vi "svfa_Process FRF (NxM).vi"(0 "stimulus signals X [EUx]":waveform(dbl)[](array[waveform]), 1 "response signals Y [EUy]":waveform(dbl)[](array[waveform]), 2 "window":T9=1 items=["None"=0, "Hanning"=1, "Hamming"=2, "Blackman-Harris"=3, "Exact Blackman"=4, "Blackman"=5, "Flat Top"=6, "4 Term B-Harris "=7, "7 Term B-Harris"=8, "Low Sidelobe"=9, "Force - Exponential"=10, "Blackman Nuttall"=11, "Triangle"=30, "Bartlett-Hanning"=31, "Bohman"=32, "Parzen"=33, "Welch"=34, "Kaiser"=60, "Dolph-Chebyshev"=61, "Gaussian"=62], 3 "force/exp settings":T8={"force window [%]"=50.0, "exp window [%]"=10.0} {"exp window [%]" min=0.0 max=100.0 format="%.2f"; "force window [%]" min=0.0 max=100.0 format="%.2f"}, 4 "averaging parameters":T12={"averaging mode"=enum."No averaging", "weighting mode"=enum."Linear", "number of averages"=10, "linear mode"=enum."Auto restart"}, 5 "error in (no error)":errorcluster, 7 "processing control":T10(ring), 9 "FRF mode":enum16{"H1", "H2", "H3"}(ring), 11 "spectra info in":T1[][](array[typedef]) {"x-axis units" items=["Time (s)"=0, "Frequency-CB (Hz)"=1, "Frequency-CPB (Hz)"=1248, "Frequency-Arbitrary (Hz)"=2357, "Quefrency (s)"=2, "Revolutions (rev)"=3, "Order"=4, "Speed (RPM)"=11, "Speed (rad/s)"=21, "Index"=65535]; "weighting filter" items=["Linear", "A-weighting", "B-weighting", "C-weighting", "ITU-R 468-4", "Dolby", "CCITT", "C-message", "Wb", "Wc", "Wd", "We", "Wf", "Wh", "Wj", "Wk", "Wm", "AES17 20 kHz lowpass", "AES17 40 kHz lowpass", "AES17 20 kHz highpass", "AES17 40 kHz highpass"]; "dB reference [EU]" format="%.2f"; "engineering units" items=["custom..."=0, "V"=1, "A"=21, "C"=30, "pC"=31, "s"=32, "-"=29, "Pa"=2, "N"=20, "g"=3, "m/s^2"=4, "m/s"=5, "m"=6, "mm/s"=12, "mm"=13, "micron/s"=14, "micron"=15, "in/s^2"=7, "in/s"=8, "in"=9, "mil/s"=10, "mil"=11, "rad/s^2"=16, "rad/s"=17, "rad"=18, "deg/s^2"=26, "deg/s"=27, "deg"=28, "RPM"=22, "cycle/s^2"=23, "Hz"=24, "cycle"=25, "strain"=19]; "spectral info"."window" items=["None "=0, "Hanning"=1, "Hamming"=2, "Blackman-Harris"=3, "Exact Blackman"=4, "Blackman"=5, "Flat Top"=6, "4 Term B-Harris "=7, "7 Term B-Harris"=8, "Low Sidelobe"=9, "Force - Exponential"=10, "Gaussian"=62]}) -> (8 "stimulus signals X [EUx] 2":waveform(dbl)[](array[waveform]), 10 "response signals Y [EUy] 2":waveform(dbl)[](array[waveform]), 12 "averages completed":dbl format="%.2f", 13 "processing control":T10(ring), 14 "complex responses [EUy/EUx]":T7(array[cluster]) {"complex spectrum" format="%.2f"; "df" format="%.2f"; "f0" format="%.2f"}, 16 "coherence":T11(array[cluster]) {"coherence" format="%.2f"; "df" format="%.2f"; "f0" format="%.2f"}, 17 "averaging done":bool, 18 "spectra info out":T1[][](array[typedef]) {"x-axis units" items=["Time (s)"=0, "Frequency-CB (Hz)"=1, "Frequency-CPB (Hz)"=1248, "Frequency-Arbitrary (Hz)"=2357, "Quefrency (s)"=2, "Revolutions (rev)"=3, "Order"=4, "Speed (RPM)"=11, "Speed (rad/s)"=21, "Index"=65535]; "weighting filter" items=["Linear", "A-weighting", "B-weighting", "C-weighting", "ITU-R 468-4", "Dolby", "CCITT", "C-message", "Wb", "Wc", "Wd", "We", "Wf", "Wh", "Wj", "Wk", "Wm", "AES17 20 kHz lowpass", "AES17 40 kHz lowpass", "AES17 20 kHz highpass", "AES17 40 kHz highpass"]; "dB reference [EU]" format="%.2f"; "engineering units" items=["custom..."=0, "V"=1, "A"=21, "C"=30, "pC"=31, "s"=32, "-"=29, "Pa"=2, "N"=20, "g"=3, "m/s^2"=4, "m/s"=5, "m"=6, "mm/s"=12, "mm"=13, "micron/s"=14, "micron"=15, "in/s^2"=7, "in/s"=8, "in"=9, "mil/s"=10, "mil"=11, "rad/s^2"=16, "rad/s"=17, "rad"=18, "deg/s^2"=26, "deg/s"=27, "deg"=28, "RPM"=22, "cycle/s^2"=23, "Hz"=24, "cycle"=25, "strain"=19]; "spectral info"."window" items=["None "=0, "Hanning"=1, "Hamming"=2, "Blackman-Harris"=3, "Exact Blackman"=4, "Blackman"=5, "Flat Top"=6, "4 Term B-Harris "=7, "7 Term B-Harris"=8, "Low Sidelobe"=9, "Force - Exponential"=10, "Gaussian"=62]}, 19 "error out":errorcluster)   [LabVIEW 2017]
uses:
  <vilib>/addons/_NISVFA/_Shared subVIs/Controls/svc_Window [Dual FFT].ctl
  <vilib>/addons/_NISVFA/_Shared subVIs/Controls/svc_Spectrum Info.ctl
  <vilib>/addons/_NISVFA/_Shared subVIs/Controls/svc_X-Axis Units.ctl
  <vilib>/addons/_NISVFA/_Shared subVIs/Controls/svc_Spectrum Type.ctl
  <vilib>/addons/_NISVFA/_Shared subVIs/Controls/svc_Engineering Units Text Ring.ctl
  <vilib>/addons/_NISVFA/_Shared subVIs/Controls/svc_Weighting Filter Text Ring.ctl
  <vilib>/addons/_NISVFA/_Shared subVIs/Controls/svc_Complimentary Spectrum Units.ctl
  <vilib>/addons/_NISVFA/_Shared subVIs/Windowing/svfa_Scaled Time Domain Window (N Ch).vi
  <vilib>/addons/_NISVFA/_Shared subVIs/Spectrum Averaging/svfa_Average Array (complex).vi
  <vilib>/addons/_NISVFA/_Shared subVIs/Spectrum Averaging/svfa_Average Array (real).vi
  <vilib>/addons/_NISVFA/_Shared subVIs/Windowing/svfa_Scaled Time Domain Window (1 Ch).vi
  <vilib>/addons/_NISVFA/_Shared subVIs/Windowing/svfa_Scaled Time Domain Window (Array).vi
  <vilib>/Analysis/4window.llb/Force Window.vi
  <vilib>/Analysis/4window.llb/Force Window (DBL).vi
  <vilib>/Analysis/4window.llb/Exponential Window.vi
  <vilib>/Analysis/4window.llb/Exponential Window (DBL).vi
  <vilib>/Utility/error.llb/Error Cluster From Error Code.vi
  <vilib>/Analysis/0measdsp.llb/Scaled Time Domain Window.vi
  <vilib>/Analysis/0measdsp.llb/Scaled Time Domain Window (DBL).vi
  <vilib>/addons/_NISVFA/_Spectrum Processing/subVIs/svfa_Spectrum Info Window to windowTd Type Def.vi
  <vilib>/addons/_NISVFA/_Shared subVIs/Common/svc_Window Parameters.vi
  <vilib>/addons/_NISVFA/_Shared subVIs/Common/svc_Get Window Info.vi
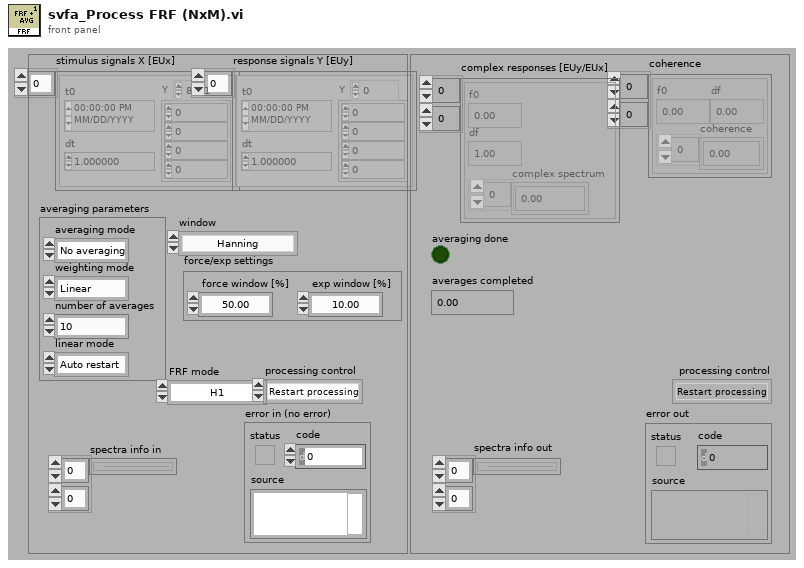
[diagram p1: front panel]
types:
  T1 = typedef "svc_Spectrum Info.ctl" = cluster{"channel name":string, "description":string, "x-axis units":T2, "spectral info":cluster{"spectrum type":T3, "linear/dB":enum16{"linear", "dB"}, "window":u16, "window size":i32, "FFT size":i32}, "engineering units":T4, "custom label":string, "dB reference [EU]":dbl, "peak units":enum16{"rms", "peak", "peak-peak"}, "weighting filter":T5, "spectral density?":bool, "unit label":string, "spectrum skewed?":bool, "complimentary spectrum units":T6}
  T2 = typedef "svc_X-Axis Units.ctl" = u16
  T3 = typedef "svc_Spectrum Type.ctl" = enum16{"FFT Spectrum [complex]", "Amplitude [Magnitude]", "Power [Magnitude^2]", "Cross Spectrum [complex]", "Frequency Response [Complex]"}
  T4 = typedef "svc_Engineering Units Text Ring.ctl" = u16
  T5 = typedef "svc_Weighting Filter Text Ring.ctl" = u16
  T6 = typedef "svc_Complimentary Spectrum Units.ctl" = enum16{"none", "radians", "degrees", "cycles", "imaginary"}
  T7 = cluster{"f0":dbl, "df":dbl, "complex spectrum":cdb[]}[][]
  T8 = cluster{"force window [%]":dbl, "exp window [%]":dbl}
  T9 = typedef "svc_Window [Dual FFT].ctl" = u32
  T10 = enum16{"Restart processing", "Continue processing", "Skip processing"}
  T11 = cluster{"f0":dbl, "df":dbl, "coherence":dbl[]}[][]
  T12 = cluster{"averaging mode":enum16{"No averaging", "Vector averaging", "RMS averaging", "Peak hold"}, "weighting mode":enum16{"Linear", "Exponential"}, "number of averages":u32, "linear mode":enum16{"One shot", "Auto restart"}}
  T13 = enum16{"No averaging", "Vector averaging", "RMS averaging", "Peak hold"}
  T14 = cluster{"f0":dbl, "df":dbl, "complex array":cdb[]}
  T15 = cluster{"f0":dbl, "df":dbl, "real FFT":dbl[]}[][]
  T16 = cluster{"f0":dbl, "df":dbl, "complex array":cdb[]}[]
  T17 = cluster{"f0":dbl, "df":dbl, "complex array":cdb[]}[][]
  T18 = cluster{"complex spectrum":cluster{"f0":dbl, "df":dbl, "complex spectrum":cdb[]}, "spectrum info":T1}
  T19 = cluster{"f0":dbl, "df":dbl, "complex spectrum":cdb[]}
  T20 = cluster{"f0":dbl, "df":dbl, "magnitude":dbl[]}[][]
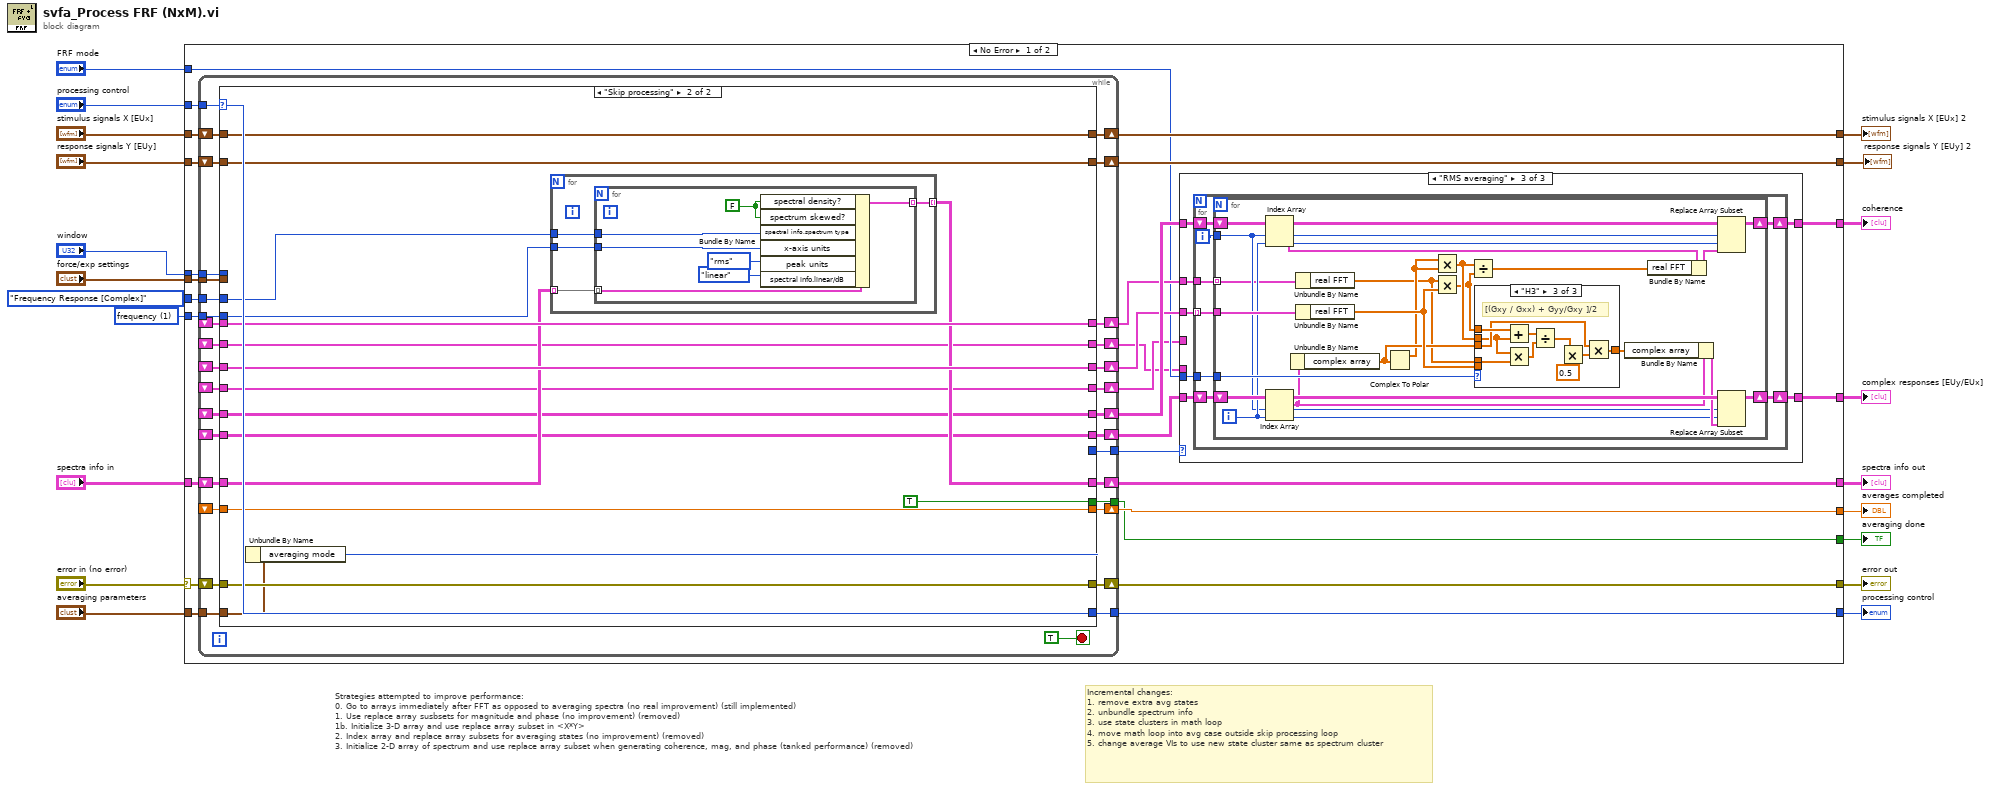
[diagram p0: block diagram]
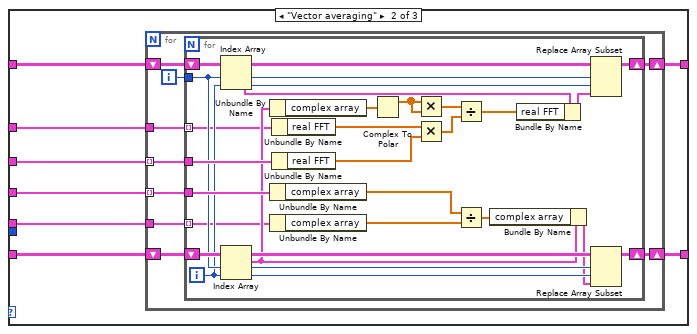
[diagram p3: hidden frame]
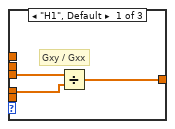
[diagram p4: hidden frame]
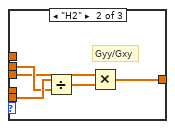
[diagram p5: hidden frame]
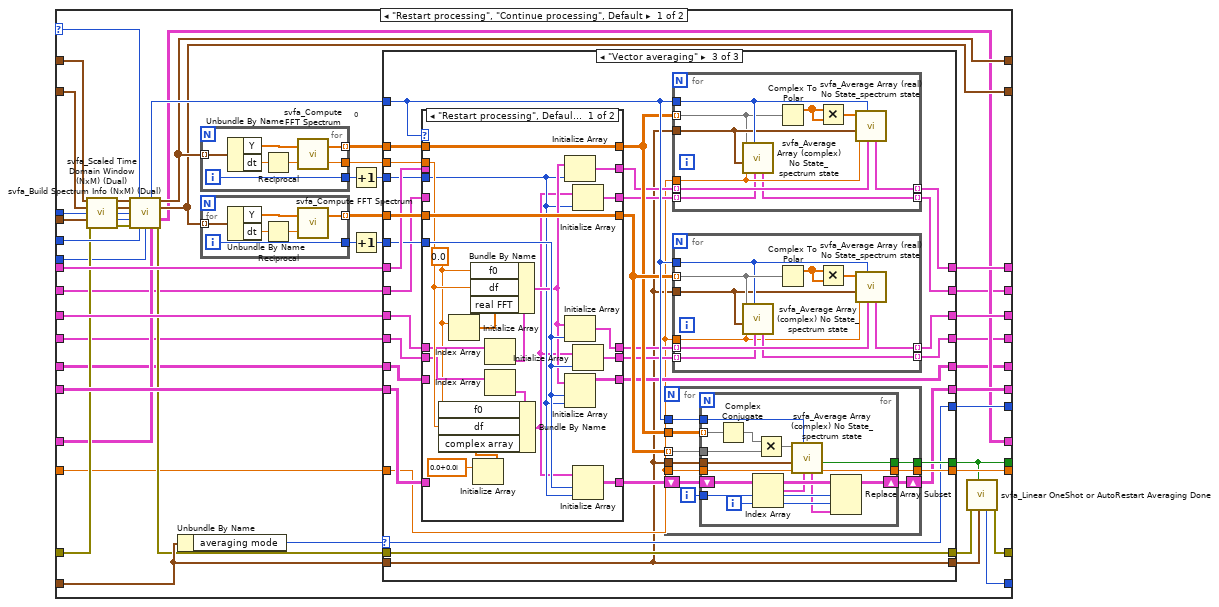
[diagram p6: hidden frame]
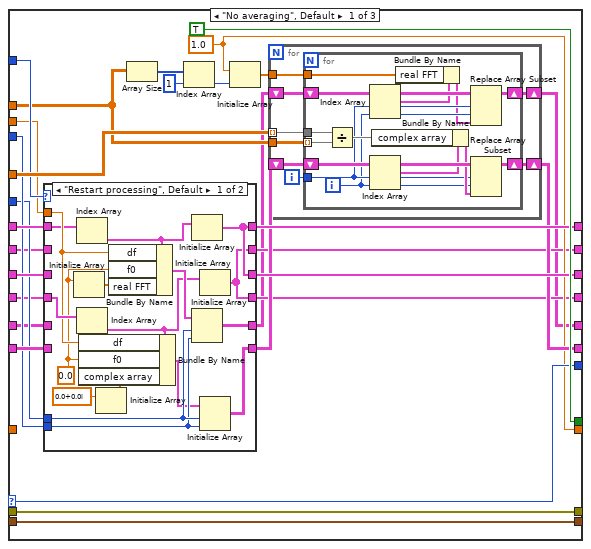
[diagram p7: hidden frame]
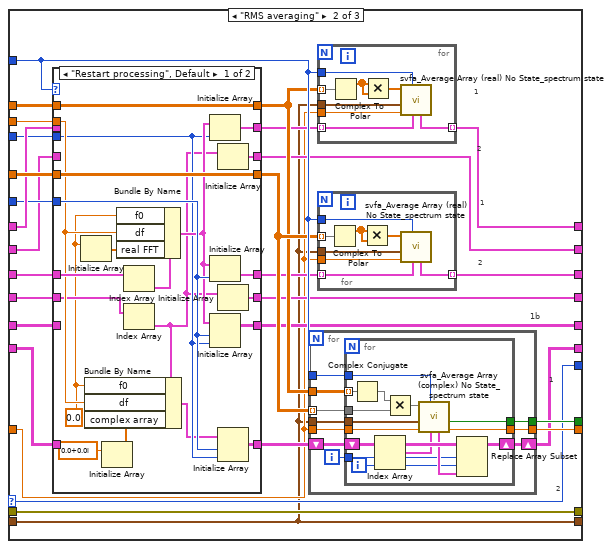
[diagram p9: hidden frame]
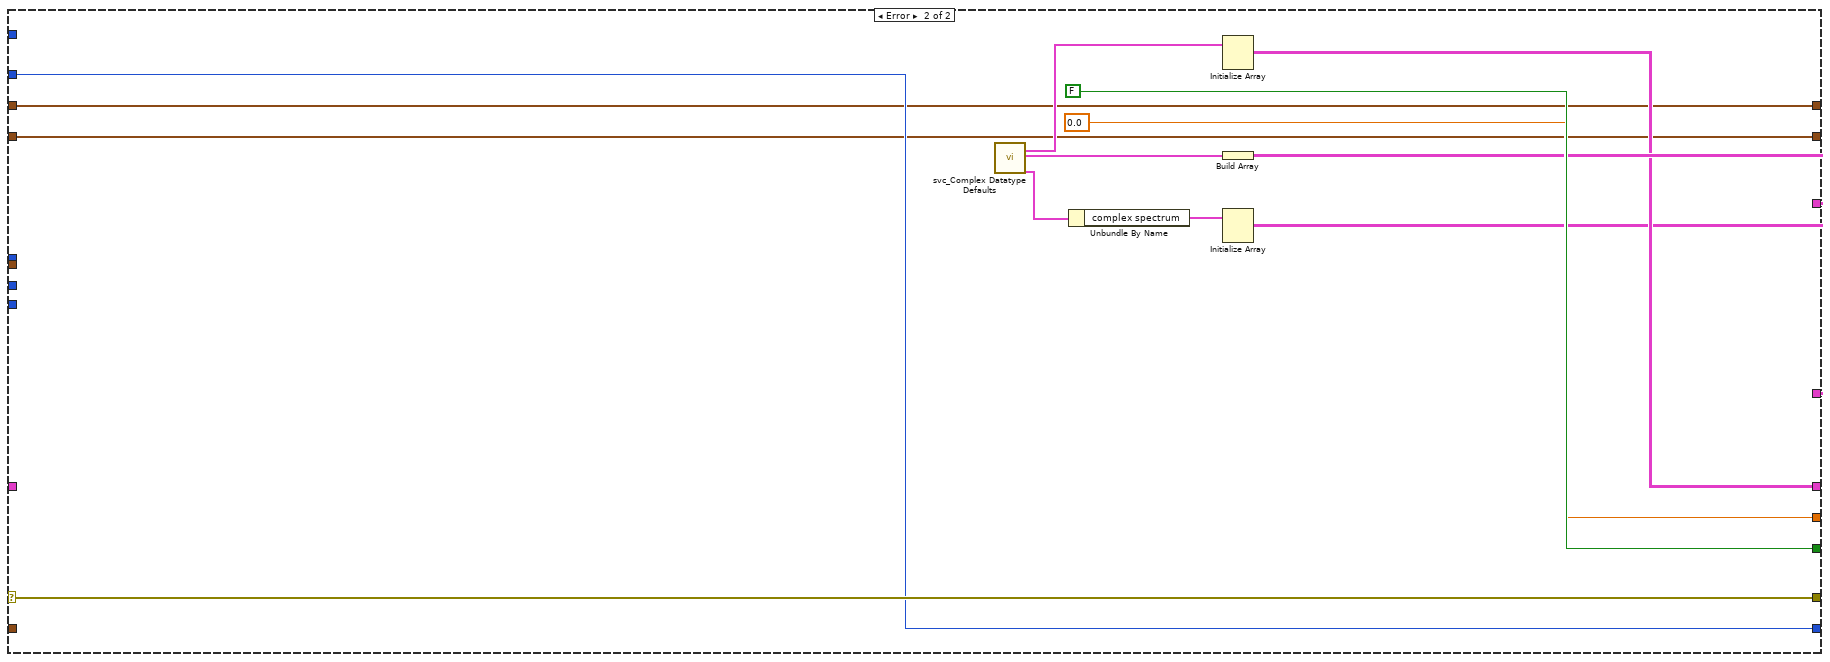
[diagram p12: hidden frame]
diagram:
  w6 = u16 1 items=["time"=0, "frequency"=1, "quefrency"=2, "revolutions"=3, "order"=4, "rpm"=11] ("x-axis units")
  # "Strategies attempted to improve performance:\n0. Go to arrays immediately after FFT as opposed to averaging spectra (no real improvement) (still implemented)\n1. Use replace array susbsets for magnitude and phase (no improvement) (removed)\n1b. Initialize 3-D array and use replace array subset in <X*Y>\n2. Index array and replace array subsets for averaging states (no improvement) (removed)\n3. Initialize 2-D array of spectrum and use replace array subset when generating coherence, mag, and phase (tanked performance) (removed)"
  # "Incremental changes:\n1. remove extra avg states\n2. unbundle spectrum info\n3. use state clusters in math loop\n4. move math loop into avg case outside skip processing loop\n5. change average VIs to use new state cluster same as spectrum cluster"
  n1 = case shown="No Error" "error in (no error)" {
    selector: "error in (no error)" -> [w44 w557]
    tunnel: [w38 w557] -> w20
    tunnel: "averaging parameters" -> [w47 _]
    tunnel: "stimulus signals X [EUx]" -> [w45 w546]
    tunnel: [w32 FALSE ("averaging done")] -> w16
    tunnel: [w46 0.0 ("averages completed")] -> w15
    tunnel: [w22 w547] -> w14
    tunnel: [w23 w552] -> w13
    tunnel: "FRF mode" -> [w26 _]
    tunnel: "processing control" -> [w43 w554]
    tunnel: [w39 w554] -> w10
    tunnel: "response signals Y [EUy]" -> [w42 w545]
    tunnel: "window" -> [w41 _]
    tunnel: "force/exp settings" -> [w40 _]
    tunnel: svc_Spectrum_Type."Frequency Response [Complex]" ("spectrum type") -> [w37 _]
    tunnel: w6 -> [w36 _]
    tunnel: [w35 w550] -> w5
    tunnel: [w34 w546] -> w4
    tunnel: [w33 w545] -> w3
    tunnel: "spectra info in" -> [w21 _]
    frame No Error {
      n2 = while {
        tunnel: [w168] -> w39
        tunnel: w40 -> [w169]
        tunnel: w41 -> [w170]
        tunnel: w43 -> [w165]
        tunnel: [w174] -> w32
        tunnel: w47 -> [w176]
        shift-right: [w164] -> w28
        shift-left: _ -> [w163]
        shift-right: [w146] -> w31
        shift-left: _ -> [w149]
        shift-right: [w162] -> w29
        shift-left: _ -> [w161]
        tunnel: w37 -> [w160]
        tunnel: w36 -> [w159]
        tunnel: [w156] -> w27
        shift-right: [w155] -> w34
        shift-left: w45 -> [w173]
        shift-right: [w154] -> w33
        shift-left: w42 -> [w171]
        shift-right: [w167] -> w38
        shift-left: w44 -> [w172]
        shift-right: [w157] -> w35
        shift-left: w21 -> [w158]
        shift-right: [w148] -> w24
        shift-left: _ -> [w151]
        shift-right: [w147] -> w25
        shift-left: _ -> [w150]
        shift-right: [w153] -> w30
        shift-left: _ -> [w152]
        shift-right: [w175] -> w46
        shift-left: _ -> [w145]
        stop <- TRUE stop-if-true
        n3 = case shown="\"Skip processing\"" w165 {
          selector: w165 -> [w177 w533]
          tunnel: w176 -> [w211 w524]
          tunnel: [w223 w520] -> w175
          tunnel: [w222 TRUE ("averaging done")] -> w174
          tunnel: w172 -> [w197 w531]
          tunnel: w171 -> [w218 w521]
          tunnel: w170 -> [w217 _]
          tunnel: w169 -> [w207 _]
          tunnel: [w214 w533] -> w168
          tunnel: [w212 w531] -> w167
          tunnel: w173 -> [w219 w522]
          tunnel: [w206 w525] -> w153
          tunnel: [w205 w530] -> w164
          tunnel: w152 -> [w204 w525]
          tunnel: w163 -> [w203 w530]
          tunnel: [w202 w529] -> w162
          tunnel: w161 -> [w201 w529]
          tunnel: w160 -> [w200 w516]
          tunnel: w159 -> [w192 w526]
          tunnel: w158 -> [w191 w528]
          tunnel: [w185 w527] -> w157
          tunnel: [w190 w523] -> w156
          tunnel: [w187 w522] -> w155
          tunnel: [w186 w521] -> w154
          tunnel: w151 -> [w184 w519]
          tunnel: w150 -> [w183 w518]
          tunnel: w149 -> [w182 w517]
          tunnel: [w181 w519] -> w148
          tunnel: [w180 w518] -> w147
          tunnel: [w179 w517] -> w146
          tunnel: w145 -> [w178 w520]
          frame "Restart processing", "Continue processing", Default {
            # "0"
            n4 = call <vilib>:"svfa_Scaled Time Domain Window (NxM) (Dual).vi"("stimulus signals X [EUx]"=w219, "response signals Y [EUy]"=w218, "window"=w217, "Force - Exponential window settings"=w207, "error in (no error)"=w197) -> ("windowed stimulus signals X [EUx]"=w221:waveform(dbl)[], "windowed response signals Y [EUy]"=w220:waveform(dbl)[], "window"=w216:T9, "window size"=w209:i32, "error out"=w208:errorcluster)  [unwired: 6 in]
            n5 = call <vilib>:"svfa_Build Spectrum Info (NxM) (Dual).vi"("stimulus signals X [EUx]"=w221, "processing control"=w177, "response signals Y [EUy]"=w220, "window"=w216, "window size"=w209, "error in (no error)"=w208, "spectrum type"=w200, "x-axis units"=w192, "spectra info in"=w191) -> ("dup processing control"=w213:T10, "dup stimulus signals X [EUx]"=w187:waveform(dbl)[], "response signals Y [EUy]"=w186:waveform(dbl)[], "spectra info out"=w185:T1[][], "error out"=w188:errorcluster)  [unwired: 2 in]
            n6 = Unbundle By Name(w211) -> ("averaging mode"=w224:T13)
            n7 = for {
              tunnel: w187 -> [w237] mode=indexing
              tunnel: [w233] -> w210 mode=indexing
              tunnel: [w232] -> w189
              tunnel: [w231] -> w196
              i -> [w231]
              n8 = Unbundle By Name ("Get Waveform Components")(w237) -> ("Y"=w236:dbl[], "dt"=w235:dbl)
              n9 = Reciprocal(x=w235) -> (1/x=w234:dbl)
              n10 = call <vilib>:"svfa_Compute FFT Spectrum.vi"("sampling frequency [Hz]"=w234, "signal [EU]"=w236) -> ("df [Hz]"=w232:dbl, "FFT spectrum [EUrms]"=w233:cdb[])
            }
            n11 = for {
              tunnel: w186 -> [w230] mode=indexing
              tunnel: [w226] -> w199 mode=indexing
              tunnel: [w225] -> w194
              i -> [w225]
              n12 = Unbundle By Name ("Get Waveform Components")(w230) -> ("Y"=w229:dbl[], "dt"=w228:dbl)
              n13 = Reciprocal(x=w228) -> (1/x=w227:dbl)
              n14 = call <vilib>:"svfa_Compute FFT Spectrum.vi"("sampling frequency [Hz]"=w227, "signal [EU]"=w229) -> ("FFT spectrum [EUrms]"=w226:cdb[])  [unwired: 1 out]
            }
            n15 = Increment(x=w196) -> (x+1=w195:i32)
            n16 = Increment(x=w194) -> (x+1=w193:i32)
            n17 = case shown="\"Vector averaging\"" w224 {
              selector: w224 -> [w252 w322 w422]
              tunnel: [w264 w321 w421] -> w198
              tunnel: w188 -> [w264 w321 w421]
              tunnel: w211 -> [w265 w313 w411]
              tunnel: [TRUE ("averaging done") w340 w441] -> w222
              tunnel: w213 -> [w262 w338 w439]
              tunnel: [w247 w339 w440] -> w223
              tunnel: [w265 w313 w411] -> w215
              tunnel: w210 -> [w250 w336 w437]
              tunnel: w199 -> [w263 w337 w438]
              tunnel: [w253 w326 w423] -> w206
              tunnel: [w257 w324 w425] -> w205
              tunnel: w204 -> [w259 w330 w432]
              tunnel: w203 -> [w260 w329 w429]
              tunnel: [w258 w325 w426] -> w202
              tunnel: w201 -> [w261 w328 w430]
              tunnel: w189 -> [w251 w323 w424]
              tunnel: w195 -> [w256 w312 w428]
              tunnel: w193 -> [w255 w327 w427]
              tunnel: [w252 w322 w422] -> w190
              tunnel: w184 -> [w241 w319 w415]
              tunnel: w183 -> [w243 w317 w414]
              tunnel: w182 -> [w244 w315 w413]
              tunnel: [w242 w320 w419] -> w181
              tunnel: [w240 w318 w417] -> w180
              tunnel: [w238 w316 w416] -> w179
              tunnel: w178 -> [_ w314 w412]
              frame "No averaging", Default {
                w247 = 1.0 ("overwrite value")
                n18 = case shown="\"Restart processing\", Default" w262 {
                  tunnel: [w276 w289] -> w258
                  tunnel: w261 -> [w274 w289]
                  tunnel: [w276 w288] -> w257
                  tunnel: w260 -> [_ w288]
                  tunnel: [w283 w287] -> w254
                  tunnel: w259 -> [_ w287]
                  tunnel: w256 -> [w277 _]
                  tunnel: w255 -> [w278 _]
                  tunnel: w251 -> [w281 _]
                  tunnel: w244 -> [_ w284]
                  tunnel: w243 -> [w282 w285]
                  tunnel: w241 -> [_ w286]
                  tunnel: [w275 w286] -> w242
                  tunnel: [w275 w285] -> w240
                  tunnel: [w279 w284] -> w239
                  frame "Restart processing", Default {
                    w272 = 0.0 ("f0")
                    n19 = Initialize Array(w272) -> (w273:dbl[])  [unwired: 1 in]
                    n20 = Index Array(array=w274) -> (element=w269:cluster{"f0":dbl, "df":dbl, "real FFT":dbl[]})  [unwired: 1 in]
                    n21 = Index Array(array=w282) -> (element=w268:T14)  [unwired: 1 in]
                    n22 = Initialize Array(cdb 0.0+0.0i ("element")) -> (w270:cdb[])  [unwired: 1 in]
                    n23 = Bundle By Name(cluster=w268, "df"=w281, "f0"=w272, "complex array"=w270) -> (w267:T14)
                    n24 = Bundle By Name(cluster=w269, "df"=w281, "f0"=w272, "real FFT"=w273) -> (w280:cluster{"f0":dbl, "df":dbl, "real FFT":dbl[]})
                    n25 = Initialize Array(w269) -> (w276:cluster{"f0":dbl, "df":dbl, "real FFT":dbl[]}[])  [unwired: 1 in]
                    n26 = Initialize Array(w280, w278, w277) -> (w279:T15)
                    n27 = Initialize Array(w268) -> (w275:T16)  [unwired: 1 in]
                    n28 = Initialize Array(w267, w278, w277) -> (w283:T17)
                  }
                  frame "Continue processing" {
                  }
                }
                n29 = Array Size(array=w250) -> (size(s)=w249:i32[])
                n30 = Index Array(array=w249, index=1) -> (element=w248:i32)
                n31 = Initialize Array(w247, w248) -> (w246:dbl[])
                n32 = for {
                  tunnel: w246 -> [w295]
                  tunnel: w250 -> [w297]
                  tunnel: w263 -> [w296] mode=indexing
                  shift-right: [w293] -> w253
                  shift-left: w254 -> [w294]
                  shift-right: [w290] -> w238
                  shift-left: w239 -> [w291]
                  i -> [w292]
                  n33 = for {
                    tunnel: w295 -> [w301]
                    tunnel: w297 -> [w305] mode=indexing
                    tunnel: w296 -> [w311]
                    shift-right: [w308] -> w293
                    shift-left: w294 -> [w309]
                    tunnel: w292 -> [w304]
                    shift-right: [w298] -> w290
                    shift-left: w291 -> [w302]
                    i -> [w303]
                    n34 = Divide(x=w311, y=w305) -> (x/y=w310:cdb[])
                    n35 = Index Array(array=w302, index (row)=w304, index (col)=w303) -> (element=w300:cluster{"f0":dbl, "df":dbl, "real FFT":dbl[]})
                    n36 = Index Array(array=w309, index (row)=w304, index (col)=w303) -> (element=w306:T14)
                    n37 = Bundle By Name(cluster=w306, "complex array"=w310) -> (w307:T14)
                    n38 = Bundle By Name(cluster=w300, "real FFT"=w301) -> (w299:cluster{"f0":dbl, "df":dbl, "real FFT":dbl[]})
                    n39 = Replace Array Subset(array=w302, new element=w299, index (row)=w304, index (col)=w303) -> (w298:T15)
                    n40 = Replace Array Subset(array=w309, new element=w307, index (row)=w304, index (col)=w303) -> (w308:T17)
                  }
                }
              }
              frame "RMS averaging" {
                # "1"
                # "1b"
                # "2"
                # "2"
                # "2"
                # "1"
                # "1"
                n41 = case shown="\"Restart processing\", Default" w338 {
                  tunnel: w337 -> [w361 w366]
                  tunnel: w336 -> [w350 w369]
                  tunnel: [w361 w366] -> w335
                  tunnel: [w350 w369] -> w334
                  tunnel: [w360 w368] -> w333
                  tunnel: [w359 w367] -> w332
                  tunnel: [w358 w365] -> w331
                  tunnel: w330 -> [_ w368]
                  tunnel: w328 -> [_ w367]
                  tunnel: w329 -> [w357 w365]
                  tunnel: w312 -> [w348 _]
                  tunnel: w327 -> [w355 _]
                  tunnel: w323 -> [w354 _]
                  tunnel: [w353 w364] -> w320
                  tunnel: w319 -> [_ w364]
                  tunnel: [w352 w363] -> w318
                  tunnel: w317 -> [w346 w363]
                  tunnel: [w351 w362] -> w316
                  tunnel: w315 -> [_ w362]
                  frame "Restart processing", Default {
                    w344 = 0.0 ("f0")
                    n42 = Initialize Array(w344) -> (w345:dbl[])  [unwired: 1 in]
                    n43 = Initialize Array(cdb 0.0+0.0i ("element")) -> (w342:cdb[])  [unwired: 1 in]
                    n44 = Index Array(array=w357) -> (element=w356:cluster{"f0":dbl, "df":dbl, "real FFT":dbl[]})  [unwired: 1 in]
                    n45 = Bundle By Name(cluster=w356, "f0"=w344, "df"=w354, "real FFT"=w345) -> (w349:cluster{"f0":dbl, "df":dbl, "real FFT":dbl[]})
                    n46 = Index Array(array=w346) -> (element=w341:T14)  [unwired: 1 in]
                    n47 = Bundle By Name(cluster=w341, "f0"=w344, "df"=w354, "complex array"=w342) -> (w347:T14)
                    n48 = Initialize Array(w349, w348) -> (w359:cluster{"f0":dbl, "df":dbl, "real FFT":dbl[]}[])
                    n49 = Initialize Array(w349, w355) -> (w358:cluster{"f0":dbl, "df":dbl, "real FFT":dbl[]}[])
                    n50 = Initialize Array(w349, w355, w348) -> (w351:T15)
                    n51 = Initialize Array(w341) -> (w353:T16)  [unwired: 1 in]
                    n52 = Initialize Array(w341) -> (w352:T16)  [unwired: 1 in]
                    n53 = Initialize Array(w347, w355, w348) -> (w360:T17)
                  }
                  frame "Continue processing", "Skip processing" {
                  }
                }
                n54 = for {
                  tunnel: w334 -> [w379]
                  tunnel: w335 -> [w378] mode=indexing
                  tunnel: w338 -> [w377]
                  tunnel: w313 -> [w376]
                  tunnel: [w375] -> w340
                  tunnel: [w374] -> w339
                  shift-right: [w372] -> w326
                  shift-left: w333 -> [w373]
                  tunnel: w314 -> [w370]
                  i -> [w371]
                  n55 = for {
                    tunnel: w377 -> [w392]
                    tunnel: w376 -> [w394]
                    tunnel: w378 -> [w389]
                    tunnel: [w391] -> w375
                    tunnel: [w390] -> w374
                    shift-right: [w387] -> w372
                    shift-left: w373 -> [w388]
                    tunnel: w371 -> [w385]
                    tunnel: w370 -> [w383]
                    tunnel: w379 -> [w380] mode=indexing
                    i -> [w382]
                    n56 = Complex Conjugate(1:w380) -> (0:w381:cdb[])
                    n57 = Index Array(array=w388, index (row)=w385, index (col)=w382) -> (element=w384:T14)
                    n58 = Multiply(x=w381, y=w389) -> (x*y=w393:cdb[])
                    n59 = call <vilib>:"svfa_Average Array (complex) No State_spectrum state.vi"("previous avg complex spectrum"=w384, "processing control"=w392, "averages completed in"=w383, "averaging parameters"=w394, "array"=w393) -> ("averages completed out"=w390:dbl, "averaging done"=w391:bool, "avg complex spectrum"=w386:T14)  [unwired: 4 in]
                    n60 = Replace Array Subset(array=w388, new element=w386, index (row)=w385, index (col)=w382) -> (w387:T17)
                  }
                }
                n61 = for {
                  tunnel: w334 -> [w407] mode=indexing
                  tunnel: w338 -> [w410]
                  tunnel: w314 -> [w405]
                  tunnel: w332 -> [w403] mode=indexing
                  tunnel: [w404] -> w325 mode=indexing
                  tunnel: w313 -> [w406]
                  n62 = Complex To Polar(r * e^(i*theta)=w407) -> (r=w409:dbl[])  [unwired: 1 out]
                  n63 = Multiply(x=w409, y=w409) -> (x*y=w408:dbl[])
                  n64 = call <vilib>:"svfa_Average Array (real) No State_spectrum state.vi"("previous avg real spectrum"=w403, "processing control"=w410, "averages completed"=w405, "averaging parameters"=w406, "array"=w408) -> ("new avg real spectrum"=w404:cluster{"f0":dbl, "df":dbl, "real FFT":dbl[]})  [unwired: 4 in, 2 out]
                }
                n65 = for {
                  tunnel: w335 -> [w399] mode=indexing
                  tunnel: w338 -> [w402]
                  tunnel: w313 -> [w401]
                  tunnel: w331 -> [w397] mode=indexing
                  tunnel: [w396] -> w324 mode=indexing
                  tunnel: w314 -> [w395]
                  n66 = Complex To Polar(r * e^(i*theta)=w399) -> (r=w400:dbl[])  [unwired: 1 out]
                  n67 = Multiply(x=w400, y=w400) -> (x*y=w398:dbl[])
                  n68 = call <vilib>:"svfa_Average Array (real) No State_spectrum state.vi"("previous avg real spectrum"=w397, "processing control"=w402, "averages completed"=w395, "averaging parameters"=w401, "array"=w398) -> ("new avg real spectrum"=w396:cluster{"f0":dbl, "df":dbl, "real FFT":dbl[]})  [unwired: 4 in, 2 out]
                }
              }
              frame "Vector averaging" {
                n69 = case shown="\"Restart processing\", Default" w439 {
                  tunnel: w438 -> [w462 w470]
                  tunnel: w437 -> [w451 w469]
                  tunnel: [w462 w470] -> w436
                  tunnel: [w451 w469] -> w435
                  tunnel: [w461 w468] -> w434
                  tunnel: [w460 w467] -> w433
                  tunnel: w432 -> [_ w468]
                  tunnel: w430 -> [_ w467]
                  tunnel: [w459 w466] -> w431
                  tunnel: w429 -> [w447 w466]
                  tunnel: w428 -> [w449 _]
                  tunnel: w427 -> [w457 _]
                  tunnel: w424 -> [w453 _]
                  tunnel: [w456 w465] -> w420
                  tunnel: [w455 w464] -> w418
                  tunnel: [w454 w463] -> w416
                  tunnel: w415 -> [_ w465]
                  tunnel: w414 -> [w446 w464]
                  tunnel: w413 -> [_ w463]
                  frame "Restart processing", Default {
                    w445 = 0.0 ("f0")
                    n70 = Initialize Array(w445) -> (w444:dbl[])  [unwired: 1 in]
                    n71 = Initialize Array(cdb 0.0+0.0i ("element")) -> (w442:cdb[])  [unwired: 1 in]
                    n72 = Index Array(array=w447) -> (element=w458:cluster{"f0":dbl, "df":dbl, "real FFT":dbl[]})  [unwired: 1 in]
                    n73 = Bundle By Name(cluster=w458, "f0"=w445, "df"=w453, "real FFT"=w444) -> (w450:cluster{"f0":dbl, "df":dbl, "real FFT":dbl[]})
                    n74 = Index Array(array=w446) -> (element=w452:T14)  [unwired: 1 in]
                    n75 = Bundle By Name(cluster=w452, "f0"=w445, "df"=w453, "complex array"=w442) -> (w448:T14)
                    n76 = Initialize Array(w450, w449) -> (w460:cluster{"f0":dbl, "df":dbl, "real FFT":dbl[]}[])
                    n77 = Initialize Array(w450, w457) -> (w459:cluster{"f0":dbl, "df":dbl, "real FFT":dbl[]}[])
                    n78 = Initialize Array(w450, w457, w449) -> (w454:T15)
                    n79 = Initialize Array(w448, w449) -> (w456:T16)
                    n80 = Initialize Array(w448, w457) -> (w455:T16)
                    n81 = Initialize Array(w448, w457, w449) -> (w461:T17)
                  }
                  frame "Continue processing", "Skip processing" {
                  }
                }
                n82 = for {
                  tunnel: w435 -> [w480]
                  tunnel: w436 -> [w479] mode=indexing
                  tunnel: w439 -> [w478]
                  tunnel: w411 -> [w477]
                  tunnel: [w476] -> w441
                  tunnel: [w475] -> w440
                  shift-right: [w473] -> w423
                  shift-left: w434 -> [w474]
                  tunnel: w412 -> [w471]
                  i -> [w472]
                  n83 = for {
                    tunnel: w478 -> [w493]
                    tunnel: w477 -> [w490]
                    tunnel: w480 -> [w489] mode=indexing
                    tunnel: w479 -> [w488]
                    tunnel: [w492] -> w476
                    tunnel: [w491] -> w475
                    tunnel: w472 -> [w487]
                    shift-right: [w482] -> w473
                    shift-left: w474 -> [w486]
                    tunnel: w471 -> [w481]
                    i -> [w485]
                    n84 = Complex Conjugate(1:w489) -> (0:w495:cdb[])
                    n85 = Index Array(array=w486, index (row)=w487, index (col)=w485) -> (element=w483:T14)
                    n86 = Multiply(x=w495, y=w488) -> (x*y=w494:cdb[])
                    n87 = call <vilib>:"svfa_Average Array (complex) No State_spectrum state.vi"("previous avg complex spectrum"=w483, "processing control"=w493, "averages completed in"=w481, "averaging parameters"=w490, "array"=w494) -> ("averages completed out"=w491:dbl, "averaging done"=w492:bool, "avg complex spectrum"=w484:T14)  [unwired: 4 in]
                    n88 = Replace Array Subset(array=w486, new element=w484, index (row)=w487, index (col)=w485) -> (w482:T17)
                  }
                }
                n89 = for {
                  tunnel: w435 -> [w506] mode=indexing
                  tunnel: w439 -> [w515]
                  tunnel: w433 -> [w511] mode=indexing
                  tunnel: [w510] -> w426 mode=indexing
                  tunnel: w420 -> [w508] mode=indexing
                  tunnel: [w507] -> w419 mode=indexing
                  tunnel: w412 -> [w512]
                  tunnel: w411 -> [w509]
                  n90 = call <vilib>:"svfa_Average Array (complex) No State_spectrum state.vi"("previous avg complex spectrum"=w508, "processing control"=w515, "averages completed in"=w512, "averaging parameters"=w509, "array"=w506) -> ("avg complex spectrum"=w507:T14)  [unwired: 4 in, 2 out]
                  n91 = Complex To Polar(r * e^(i*theta)=w506) -> (r=w514:dbl[])  [unwired: 1 out]
                  n92 = Multiply(x=w514, y=w514) -> (x*y=w513:dbl[])
                  n93 = call <vilib>:"svfa_Average Array (real) No State_spectrum state.vi"("previous avg real spectrum"=w511, "processing control"=w515, "averages completed"=w512, "averaging parameters"=w509, "array"=w513) -> ("new avg real spectrum"=w510:cluster{"f0":dbl, "df":dbl, "real FFT":dbl[]})  [unwired: 4 in, 2 out]
                }
                n94 = for {
                  tunnel: w436 -> [w505] mode=indexing
                  tunnel: w439 -> [w503]
                  tunnel: w411 -> [w496]
                  tunnel: [w504] -> w425 mode=indexing
                  tunnel: w431 -> [w500] mode=indexing
                  tunnel: w418 -> [w499] mode=indexing
                  tunnel: [w498] -> w417 mode=indexing
                  tunnel: w412 -> [w497]
                  n95 = call <vilib>:"svfa_Average Array (complex) No State_spectrum state.vi"("previous avg complex spectrum"=w499, "processing control"=w503, "averages completed in"=w497, "averaging parameters"=w496, "array"=w505) -> ("avg complex spectrum"=w498:T14)  [unwired: 4 in, 2 out]
                  n96 = Complex To Polar(r * e^(i*theta)=w505) -> (r=w502:dbl[])  [unwired: 1 out]
                  n97 = Multiply(x=w502, y=w502) -> (x*y=w501:dbl[])
                  n98 = call <vilib>:"svfa_Average Array (real) No State_spectrum state.vi"("previous avg real spectrum"=w500, "processing control"=w503, "averages completed"=w497, "averaging parameters"=w496, "array"=w501) -> ("new avg real spectrum"=w504:cluster{"f0":dbl, "df":dbl, "real FFT":dbl[]})  [unwired: 4 in, 2 out]
                }
              }
            }
            n99 = call <vilib>:"svfa_Linear OneShot or AutoRestart Averaging Done.vi"("averaging parameters"=w215, "averaging done"=w222, "error in (no error)"=w198) -> ("error out"=w212:errorcluster, "processing control"=w214:T10)  [unwired: 7 in]
          }
          frame "Skip processing" {
            n100 = Unbundle By Name(w524) -> ("averaging mode"=w523:T13)
            n101 = for {
              tunnel: w528 -> [w537] mode=indexing
              tunnel: [w536] -> w527 mode=indexing
              tunnel: w526 -> [w535]
              tunnel: w516 -> [w534]
              n102 = for {
                tunnel: w537 -> [w541] mode=indexing
                tunnel: [w540] -> w536 mode=indexing
                tunnel: w535 -> [w539]
                tunnel: w534 -> [w538]
                w543 = FALSE ("spectral density?")
                n103 = Bundle By Name(cluster=w541, "spectral density?"=w543, "spectrum skewed?"=w543, "spectral info.spectrum type"=w538, "x-axis units"=w539, "peak units"=enum16{"rms", "peak", "peak-peak"}."rms", "spectral info.linear/dB"=enum16{"linear", "dB"}."linear") -> (w540:T1)
              }
            }
          }
        }
      }
      n104 = case shown="\"RMS averaging\"" w27 {
        tunnel: w30 -> [w48 w57 w95]
        tunnel: w28 -> [_ w56 w96]
        tunnel: w29 -> [_ w55 w97]
        tunnel: [w49 w51 w93] -> w23
        tunnel: [w48 w50 w94] -> w22
        tunnel: w26 -> [_ _ w92]
        tunnel: w31 -> [w49 w52 w91]
        tunnel: w24 -> [_ w54 _]
        tunnel: w25 -> [_ w53 _]
        frame "No averaging", Default {
        }
        frame "Vector averaging" {
          n105 = for {
            tunnel: w55 -> [w66]
            tunnel: w56 -> [w65] mode=indexing
            tunnel: w53 -> [w63] mode=indexing
            tunnel: w54 -> [w62]
            shift-right: [w59] -> w51
            shift-left: w52 -> [w61]
            shift-right: [w58] -> w50
            shift-left: w57 -> [w64]
            i -> [w60]
            n106 = for {
              tunnel: w66 -> [w70] mode=indexing
              tunnel: w65 -> [w88]
              tunnel: w63 -> [w85]
              tunnel: w62 -> [w67] mode=indexing
              shift-right: [w75] -> w59
              shift-left: w61 -> [w79]
              shift-right: [w82] -> w58
              shift-left: w64 -> [w83]
              tunnel: w60 -> [w81]
              i -> [w80]
              n107 = Index Array(array=w79, index (row)=w81, index (col)=w80) -> (element=w78:cluster{"f0":dbl, "df":dbl, "real FFT":dbl[]})
              n108 = Index Array(array=w83, index (row)=w81, index (col)=w80) -> (element=w73:T14)
              n109 = Unbundle By Name(w73) -> ("complex array"=w86:cdb[])
              n110 = Unbundle By Name(w85) -> ("complex array"=w84:cdb[])
              n111 = Unbundle By Name(w67) -> ("complex array"=w68:cdb[])
              n112 = Unbundle By Name(w70) -> ("real FFT"=w69:dbl[])
              n113 = Unbundle By Name(w88) -> ("real FFT"=w87:dbl[])
              n114 = Complex To Polar(r * e^(i*theta)=w86) -> (r=w71:dbl[])  [unwired: 1 out]
              n115 = Multiply(x=w71, y=w71) -> (x*y=w90:dbl[])
              n116 = Multiply(x=w69, y=w87) -> (x*y=w89:dbl[])
              n117 = Divide(x=w90, y=w89) -> (x/y=w76:dbl[])
              n118 = Divide(x=w84, y=w68) -> (x/y=w72:cdb[])
              n119 = Bundle By Name(cluster=w73, "complex array"=w72) -> (w74:T14)
              n120 = Bundle By Name(cluster=w78, "real FFT"=w76) -> (w77:cluster{"f0":dbl, "df":dbl, "real FFT":dbl[]})
              n121 = Replace Array Subset(array=w79, new element=w77, index (row)=w81, index (col)=w80) -> (w75:T15)
              n122 = Replace Array Subset(array=w83, new element=w74, index (row)=w81, index (col)=w80) -> (w82:T17)
            }
          }
        }
        frame "RMS averaging" {
          n123 = for {
            tunnel: w97 -> [w102]
            tunnel: w96 -> [w101] mode=indexing
            tunnel: w92 -> [w100]
            shift-right: [w105] -> w93
            shift-left: w91 -> [w99]
            shift-right: [w104] -> w94
            shift-left: w95 -> [w103]
            i -> [w98]
            n124 = for {
              tunnel: w102 -> [w107] mode=indexing
              tunnel: w101 -> [w126]
              tunnel: w100 -> [w125]
              shift-right: [w122] -> w105
              shift-left: w99 -> [w123]
              shift-right: [w114] -> w104
              shift-left: w103 -> [w118]
              tunnel: w98 -> [w115]
              i -> [w116]
              n125 = Index Array(array=w123, index (row)=w115, index (col)=w116) -> (element=w121:cluster{"f0":dbl, "df":dbl, "real FFT":dbl[]})
              n126 = Index Array(array=w118, index (row)=w115, index (col)=w116) -> (element=w113:T14)
              n127 = Unbundle By Name(w113) -> ("complex array"=w112:cdb[])
              n128 = Unbundle By Name(w107) -> ("real FFT"=w108:dbl[])
              n129 = Unbundle By Name(w126) -> ("real FFT"=w124:dbl[])
              n130 = Complex To Polar(r * e^(i*theta)=w112) -> (r=w109:dbl[])  [unwired: 1 out]
              n131 = Multiply(x=w109, y=w109) -> (x*y=w110:dbl[])
              n132 = Multiply(x=w108, y=w124) -> (x*y=w106:dbl[])
              n133 = Divide(x=w110, y=w106) -> (x/y=w120:dbl[])
              n134 = case shown="\"H3\"" w125 {
                tunnel: [w129 w130 w142] -> w111
                tunnel: w108 -> [w128 _ w138]
                tunnel: w124 -> [_ w134 _]
                tunnel: w112 -> [w127 w131 w136]
                tunnel: w110 -> [_ w133 w135]
                tunnel: w106 -> [_ _ w141]
                frame "H1", Default {
                  # "Gxy / Gxx"
                  n135 = Divide(x=w127, y=w128) -> (x/y=w129:cdb[])
                }
                frame "H2" {
                  # "Gyy/Gxy"
                  n136 = Divide(x=w134, y=w133) -> (x/y=w132:dbl[])
                  n137 = Multiply(x=w131, y=w132) -> (x*y=w130:cdb[])
                }
                frame "H3" {
                  # "[(Gxy / Gxx) + Gyy/Gxy ]/2"
                  n138 = Add(x=w141, y=w135) -> (x+y=w140:dbl[])
                  n139 = Multiply(x=w135, y=w138) -> (x*y=w137:dbl[])
                  n140 = Divide(x=w140, y=w137) -> (x/y=w139:dbl[])
                  n141 = Multiply(x=w139, y=0.5) -> (x*y=w143:dbl[])
                  n142 = Multiply(x=w136, y=w143) -> (x*y=w142:cdb[])
                }
              }
              n143 = Bundle By Name(cluster=w113, "complex array"=w111) -> (w117:T14)
              n144 = Bundle By Name(cluster=w121, "real FFT"=w120) -> (w119:cluster{"f0":dbl, "df":dbl, "real FFT":dbl[]})
              n145 = Replace Array Subset(array=w123, new element=w119, index (row)=w115, index (col)=w116) -> (w122:T15)
              n146 = Replace Array Subset(array=w118, new element=w117, index (row)=w115, index (col)=w116) -> (w114:T17)
            }
          }
        }
      }
    }
    frame Error {
      n147 = call <vilib>:"svc_Complex Datatype Defaults.vi"() -> ("dead spectrum info"=w551:T1, "empty array of spectra"=w553:cluster{"f0":dbl, "df":dbl, "magnitude":dbl[]}[], "complex spectrum"=w549:T18)  [unwired: 11 in, 6 out]
      n148 = Unbundle By Name(w549) -> ("complex spectrum"=w548:T19)
      n149 = Initialize Array(w551) -> (w550:T1[][])  [unwired: 2 in]
      n150 = Build Array(w553) -> (w552:T20)
      n151 = Initialize Array(w548) -> (w547:T7)  [unwired: 2 in]
    }
  }
  "error out" <- w20
  "averages completed" <- w15
  "averaging done" <- w16
  "complex responses [EUy/EUx]" <- w14
  "coherence" <- w13
  "processing control" <- w10
  "spectra info out" <- w5
  "stimulus signals X [EUx] 2" <- w4
  "response signals Y [EUy] 2" <- w3
